vi "Configure Mirror.vi"(7 "mirror index (0)":u8, 8 "error in (no error)":errorcluster, 10 "mirror position index":u8, 11 "SOL MS in":refnum<class "PL SOL Instruments MS.lvclass">) -> (0 "error out":errorcluster, 3 "SOL MS out":refnum<class "PL SOL Instruments MS.lvclass">)   [LabVIEW 2015, in "PL SOL Instruments MS.lvclass"]
doc: "Configures mirror."
uses:
  PL SOL Instruments MS.lvclass
  PL SOL Instruments MS.lvclass/PL SOL Instruments MS.ctl
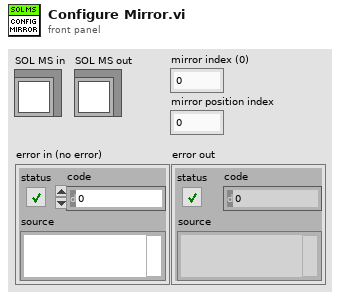
[diagram p1: front panel]
types:
  T1 = cluster{"name":string, "step timeout, ms":u32, "reset timeout, ms":u32, "positions":cluster{"name":string, "position":i32}[], "current position index":u8}[]
  T2 = cluster{"name":string, "step timeout, ms":u32, "reset timeout, ms":u32, "positions":cluster{"name":string, "position":i32}[], "current position index":u8}
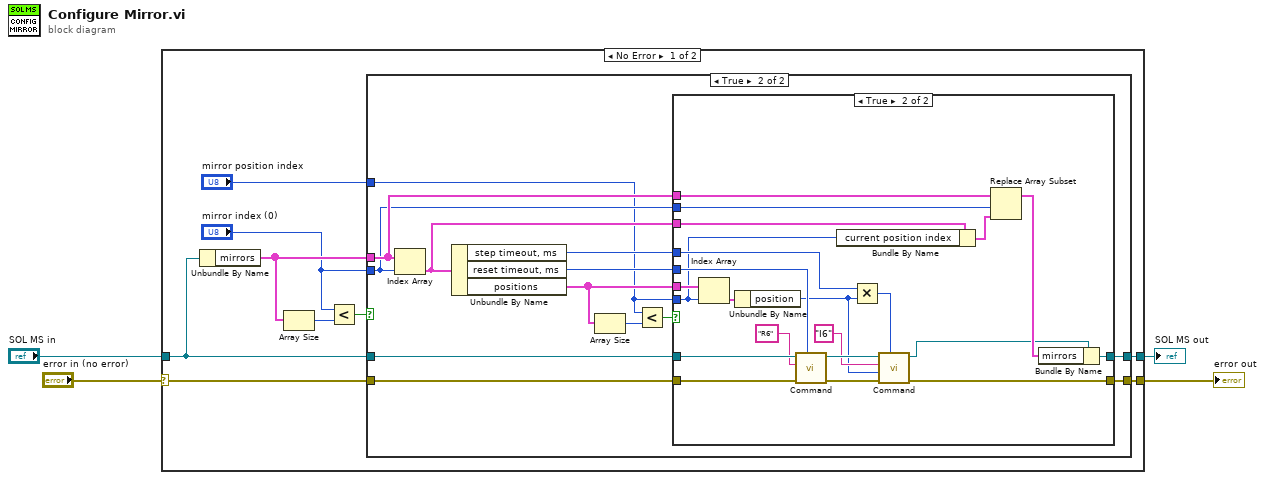
[diagram p0: block diagram]
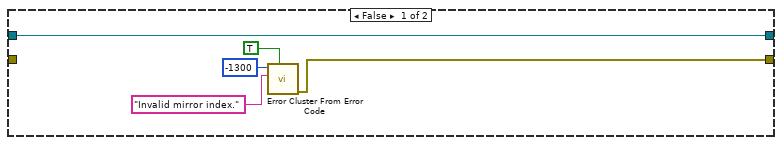
[diagram p2: hidden frame]
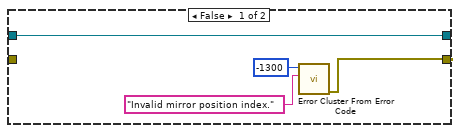
[diagram p3: hidden frame]
diagram:
  n1 = case shown="No Error" "error in (no error)" {
    selector: "error in (no error)" -> [w7 w57]
    tunnel: "SOL MS in" -> [w13 w58]
    tunnel: [w6 w58] -> w3
    tunnel: [w5 w57] -> w2
    frame No Error {
      n2 = Unbundle By Name(w13) -> ("mirrors"=w12:T1)
      n3 = Array Size(array=w12) -> (size(s)=w10:i32)
      n4 = Less?(x="mirror index (0)", y=w10) -> (x < y?=w9:bool)
      n5 = case shown="True" w9 {
        tunnel: w7 -> [_ w23]
        tunnel: w13 -> [w18 w24]
        tunnel: [w18 w31] -> w6
        tunnel: [w17 w30] -> w5
        tunnel: w12 -> [_ w26]
        tunnel: "mirror position index" -> [_ w20]
        tunnel: "mirror index (0)" -> [_ w21]
        frame False {
          n6 = call <vilib>:"Error Cluster From Error Code.vi"("show call chain? (False)"=TRUE, "error message (\"\")"="Invalid mirror index." ("error message (\"\")"), "error code (0)"=-1300) -> ("error out"=w17:errorcluster)  [unwired: 6 in]
        }
        frame True {
          n7 = Index Array(array=w26, index=w21) -> (element=w25:T2)
          n8 = Unbundle By Name(w25) -> ("step timeout, ms"=w27:u32, "reset timeout, ms"=w28:u32, "positions"=w29:cluster{"name":string, "position":i32}[])
          n9 = Array Size(array=w29) -> (size(s)=w19:i32)
          n10 = Less?(x=w20, y=w19) -> (x < y?=w22:bool)
          n11 = case shown="True" w22 {
            tunnel: w23 -> [_ w46]
            tunnel: w24 -> [w35 w56]
            tunnel: [w35 w55] -> w31
            tunnel: [w34 w54] -> w30
            tunnel: w29 -> [_ w48]
            tunnel: w20 -> [_ w47]
            tunnel: w28 -> [_ w49]
            tunnel: w27 -> [_ w50]
            tunnel: w26 -> [_ w53]
            tunnel: w25 -> [_ w52]
            tunnel: w21 -> [_ w51]
            frame False {
              n12 = call <vilib>:"Error Cluster From Error Code.vi"("error message (\"\")"="Invalid mirror position index." ("error message (\"\")"), "error code (0)"=-1300) -> ("error out"=w34:errorcluster)  [unwired: 7 in]
            }
            frame True {
              n13 = Index Array(array=w48, index=w47) -> (element=w45:cluster{"name":string, "position":i32})
              n14 = Unbundle By Name(w45) -> ("position"=w37:i32)
              n15 = call "Command.vi"("additional timeout, ms (0)"=w49, "error in (no error)"=w46, "command"="R6", "SOL MS in"=w56) -> ("error out"=w40:errorcluster, "SOL MS out"=w39:refnum<class "PL SOL Instruments MS.lvclass">)  [unwired: 6 in]
              n16 = Bundle By Name(cluster=w52, "current position index"=w47) -> (w44:T2)
              n17 = Multiply(x=w50, y=w37) -> (x*y=w42:u32)
              n18 = call "Command.vi"("additional timeout, ms (0)"=w42, "error in (no error)"=w40, "data"=w37, "command"="I6", "SOL MS in"=w39) -> ("error out"=w54:errorcluster, "SOL MS out"=w41:refnum<class "PL SOL Instruments MS.lvclass">)  [unwired: 5 in]
              n19 = Replace Array Subset(array=w53, new element=w44, index=w51) -> (w43:T1)
              n20 = Bundle By Name(cluster=w41, "mirrors"=w43) -> (w55:refnum<class "PL SOL Instruments MS.lvclass">)
            }
          }
        }
      }
    }
    frame Error {
    }
  }
  "SOL MS out" <- w3
  "error out" <- w2
